vi "Attenuator Convert Stimulus Cluster.vi"(4 "Conversion":enum16{"Cluster - HTML", "HTML - Cluster"}(ring), 6 "Stimulus Key Array In":T6, 7 "Stimulus Cluster In":T1={"ATT Stimulus"={"Normalize"=FALSE, "Value (dB)"=0.0}, "VNA Stimulus"={"Use Instrument Settings"=FALSE, "Blank Frequencies"=FALSE, "Sweep Type"=enum."Linear", "Sweep"={"Fstart"=500.0, "Fstop"=1500.0, "Units"=enum."MHz", "Points"=201}, "Power (dBm)"=999.0, "IFBW (Hz)"=-1.0, "Sweep Time (s)"=-1.0, "Calibration"={"State"=FALSE, "String"=""}}} {"VNA Stimulus"."Sweep Time (s)" format="%.3g"}) -> (1 "Stimulus Cluster Out":T1={"ATT Stimulus"={"Normalize"=FALSE, "Value (dB)"=0.0}, "VNA Stimulus"={"Use Instrument Settings"=FALSE, "Blank Frequencies"=FALSE, "Sweep Type"=enum."Linear", "Sweep"={"Fstart"=500.0, "Fstop"=1500.0, "Units"=enum."MHz", "Points"=201}, "Power (dBm)"=999.0, "IFBW (Hz)"=-1.0, "Sweep Time (s)"=-1.0, "Calibration"={"State"=FALSE, "String"=""}}} {"VNA Stimulus"."Sweep Time (s)" format="%.3g"}, 2 "Stumulus HTML Out":string)   [LabVIEW 2011]
uses:
  ITK EXT/utils/keyedarr.llb/Keyed Array.ctl
  TypeDefs/Attenuator Stimulus Parameters.ctl
  TypeDefs/Attenuator ATT Stimulus.ctl
  TypeDefs/Attenuator VNA Stimulus.ctl
  S Parameter/TypeDefs/SP Frequency Units.ctl
  TypeDefs/Attenuator VNA Calibration State.ctl
  ITK EXT/utils/strutil.llb/Case Matching.ctl
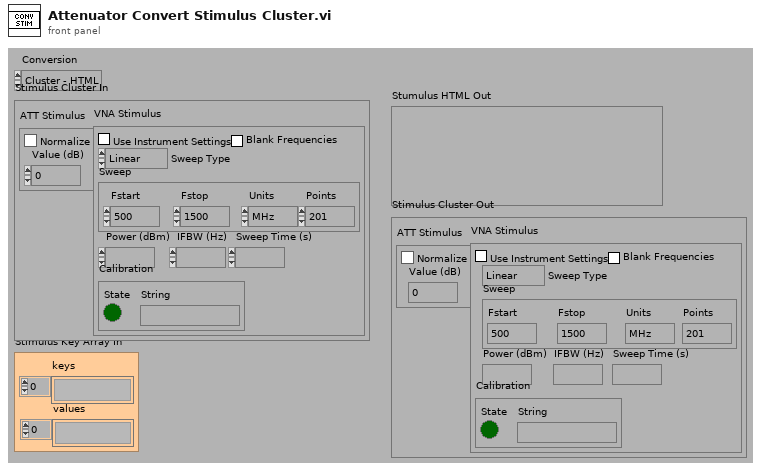
[diagram p1: front panel]
types:
  T1 = typedef "Attenuator Stimulus Parameters.ctl" = cluster{"ATT Stimulus":T2, "VNA Stimulus":T3}
  T2 = typedef "Attenuator ATT Stimulus.ctl" = cluster{"Normalize":bool, "Value (dB)":dbl}
  T3 = typedef "Attenuator VNA Stimulus.ctl" = cluster{"Use Instrument Settings":bool, "Blank Frequencies":bool, "Sweep Type":enum32{"Linear", "Logarithmic", "List", "Power", "CW"}, "Sweep":cluster{"Fstart":dbl, "Fstop":dbl, "Units":T4, "Points":i32}, "Power (dBm)":dbl, "IFBW (Hz)":dbl, "Sweep Time (s)":dbl, "Calibration":T5}
  T4 = typedef "SP Frequency Units.ctl" = enum16{"Hz", "kHz", "MHz", "GHz", "Points"}
  T5 = typedef "Attenuator VNA Calibration State.ctl" = cluster{"State":bool, "String":string}
  T6 = typedef "Keyed Array.ctl" = cluster{"keys":string[], "values":string[]}
  T7 = typedef "Case Matching.ctl" = enum16{"a != A", "a == A", "system"}
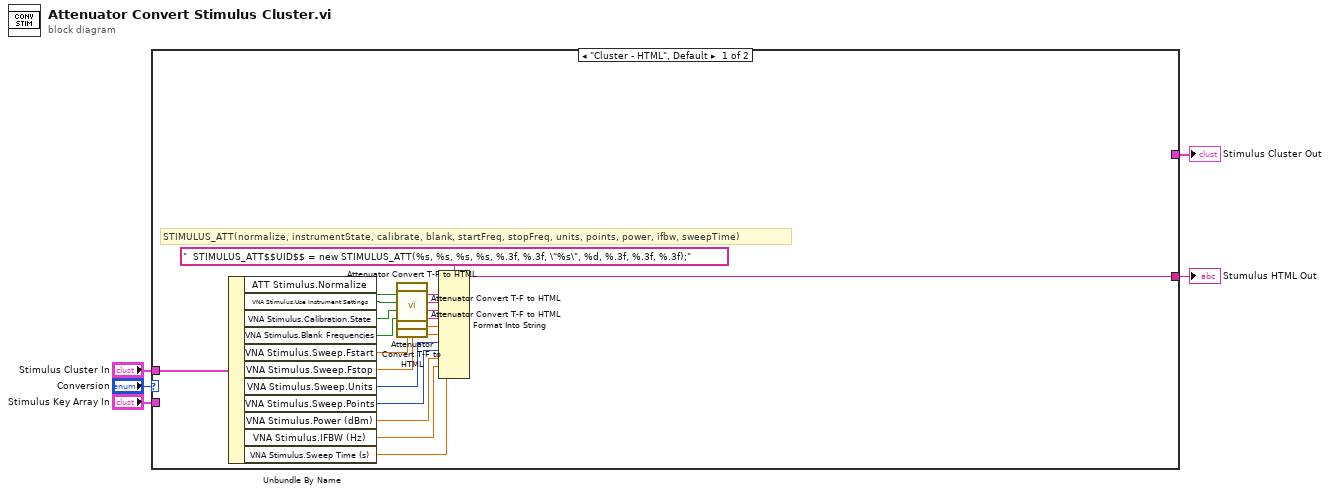
[diagram p0: block diagram]
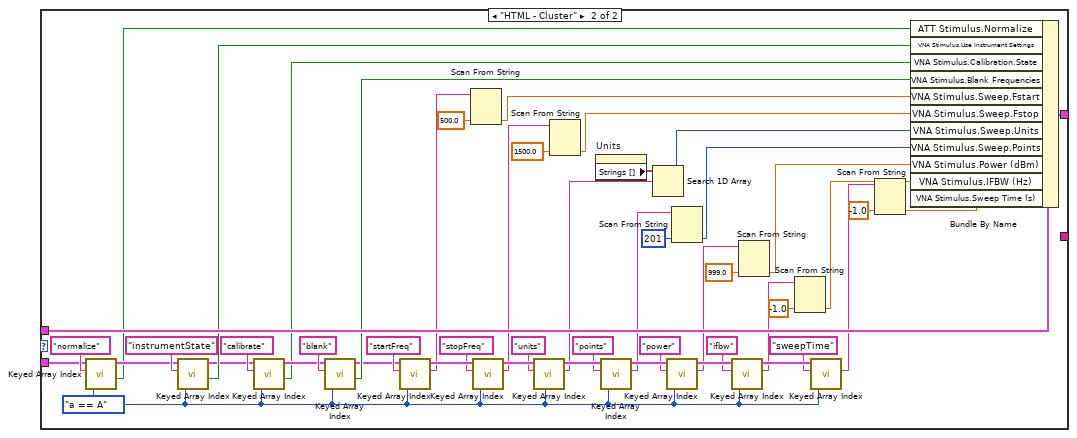
[diagram p2: hidden frame]
diagram:
  n1 = case shown="\"Cluster - HTML\", Default" "Conversion" {
    tunnel: "Stimulus Cluster In" -> [w23 w58]
    tunnel: "Stimulus Key Array In" -> [_ w27]
    tunnel: [w18 _] -> w1
    tunnel: [_ w40] -> w2
    frame "Cluster - HTML", Default {
      # "STIMULUS_ATT(normalize, instrumentState, calibrate, blank, startFreq, stopFreq, units, points, power, ifbw, sweepTime)"
      n2 = Unbundle By Name(w23) -> ("ATT Stimulus.Normalize"=w8:bool, "VNA Stimulus.Use Instrument Settings"=w6:bool, "VNA Stimulus.Calibration.State"=w9:bool, "VNA Stimulus.Blank Frequencies"=w15:bool, "VNA Stimulus.Sweep.Fstart"=w12:dbl, "VNA Stimulus.Sweep.Fstop"=w11:dbl, "VNA Stimulus.Sweep.Units"=w13:T4, "VNA Stimulus.Sweep.Points"=w22:i32, "VNA Stimulus.Power (dBm)"=w21:dbl, "VNA Stimulus.IFBW (Hz)"=w20:dbl, "VNA Stimulus.Sweep Time (s)"=w19:dbl)
      n3 = call "Attenuator Convert T-F to HTML.vi"("(T/F)"=w8) -> ("HTML (true/false)"=w16:string)  [unwired: 10 in]
      n4 = call "Attenuator Convert T-F to HTML.vi"("(T/F)"=w6) -> ("HTML (true/false)"=w7:string)  [unwired: 10 in]
      n5 = call "Attenuator Convert T-F to HTML.vi"("(T/F)"=w9) -> ("HTML (true/false)"=w10:string)  [unwired: 10 in]
      n6 = call "Attenuator Convert T-F to HTML.vi"("(T/F)"=w15) -> ("HTML (true/false)"=w14:string)  [unwired: 10 in]
      n7 = Format Into String(format string="  STIMULUS_ATT$$UID$$ = new STIMULUS_ATT(%s, %s, %s, %s, %.3f, %.3f, \"%s\", %d, %.3f, %.3f, %.3f);", w16, w7, w10, w14, w12, w11, w13, w22, w21, w20, w19) -> (resulting string=w18:string)  [unwired: 2 in, 1 out]
    }
    frame "HTML - Cluster" {
      w25 = Case_Matching."a == A" ("case matching (sensitive)")
      n8 = call "Keyed Array Index.vi"("case matching (sensitive)"=w25, "key"="normalize", "array in"=w27) -> ("valid key"=w24:bool, "duplicate array"=w26:T6)  [unwired: 1 in, 2 out]
      n9 = call "Keyed Array Index.vi"("case matching (sensitive)"=w25, "key"="instrumentState", "array in"=w26) -> ("valid key"=w34:bool, "duplicate array"=w32:T6)  [unwired: 1 in, 2 out]
      n10 = call "Keyed Array Index.vi"("case matching (sensitive)"=w25, "key"="calibrate", "array in"=w32) -> ("valid key"=w30:bool, "duplicate array"=w31:T6)  [unwired: 1 in, 2 out]
      n11 = call "Keyed Array Index.vi"("case matching (sensitive)"=w25, "key"="blank", "array in"=w31) -> ("valid key"=w57:bool, "duplicate array"=w29:T6)  [unwired: 1 in, 2 out]
      n12 = call "Keyed Array Index.vi"("case matching (sensitive)"=w25, "key"="startFreq", "array in"=w29) -> ("value"=w56:string, "duplicate array"=w72:T6)  [unwired: 1 in, 2 out]
      n13 = Scan From String(input string=w56, default 1=500.0 ("default value 1")) -> (output 1=w36:dbl)  [unwired: 3 in, 3 out]
      n14 = call "Keyed Array Index.vi"("case matching (sensitive)"=w25, "key"="stopFreq", "array in"=w72) -> ("value"=w53:string, "duplicate array"=w71:T6)  [unwired: 1 in, 2 out]
      n15 = call "Keyed Array Index.vi"("case matching (sensitive)"=w25, "key"="units", "array in"=w71) -> ("value"=w37:string, "duplicate array"=w70:T6)  [unwired: 1 in, 2 out]
      n16 = Scan From String(input string=w53, default 1=1500.0 ("default value 1")) -> (output 1=w35:dbl)  [unwired: 3 in, 3 out]
      n17 = property on="Units" class="Enum (strict)"() -> ("Strings []"=w38:string[])  [unwired: 2 in, 2 out]
      n18 = call "Keyed Array Index.vi"("case matching (sensitive)"=w25, "key"="points", "array in"=w70) -> ("value"=w51:string, "duplicate array"=w69:T6)  [unwired: 1 in, 2 out]
      n19 = Search 1D Array(1D array=w38, element=w37) -> (index of element=w39:i32)  [unwired: 1 out]
      n20 = call "Keyed Array Index.vi"("case matching (sensitive)"=w25, "key"="power", "array in"=w69) -> ("value"=w48:string, "duplicate array"=w68:T6)  [unwired: 1 in, 2 out]
      n21 = Scan From String(input string=w51, default 1=201 ("default value 1")) -> (output 1=w50:i32)  [unwired: 3 in, 3 out]
      n22 = call "Keyed Array Index.vi"("case matching (sensitive)"=w25, "key"="ifbw", "array in"=w68) -> ("value"=w44:string, "duplicate array"=w67:T6)  [unwired: 1 in, 2 out]
      n23 = Scan From String(input string=w48, default 1=999.0 ("default value 1")) -> (output 1=w47:dbl)  [unwired: 3 in, 3 out]
      n24 = Scan From String(input string=w44, default 1=-1.0 ("default value 1")) -> (output 1=w43:dbl)  [unwired: 3 in, 3 out]
      n25 = call "Keyed Array Index.vi"("case matching (sensitive)"=w25, "key"="sweepTime", "array in"=w67) -> ("value"=w42:string)  [unwired: 1 in, 3 out]
      n26 = Scan From String(input string=w42, default 1=-1.0 ("default value 1")) -> (output 1=w41:dbl)  [unwired: 3 in, 3 out]
      n27 = Bundle By Name(cluster=w58, "ATT Stimulus.Normalize"=w24, "VNA Stimulus.Use Instrument Settings"=w34, "VNA Stimulus.Calibration.State"=w30, "VNA Stimulus.Blank Frequencies"=w57, "VNA Stimulus.Sweep.Fstart"=w36, "VNA Stimulus.Sweep.Fstop"=w35, "VNA Stimulus.Sweep.Units"=w39, "VNA Stimulus.Sweep.Points"=w50, "VNA Stimulus.Power (dBm)"=w47, "VNA Stimulus.IFBW (Hz)"=w43, "VNA Stimulus.Sweep Time (s)"=w41) -> (w40:T1)
    }
  }
  "Stumulus HTML Out" <- w1
  "Stimulus Cluster Out" <- w2
